vi "Zadanie 3.vi"() -> ()   [LabVIEW 2020]
doc: "Use this template to build a producer/consumer design pattern with events to produce queue items. Use this design pattern instead of the User Interface Event Handler pattern for user interfaces when you want to execute code asynchronously in response to an event without slowing the user interface responsiveness."
panel:
  out "Waveform Graph":dbl[](graph)
  in  "What to add?":dbl
  out "Busy":bool
  in  "?":bool
  out "Generated numbers":dbl[](array[numeric])
  in  "?":bool
  in  "REMOVE":bool
  in  "stop":bool
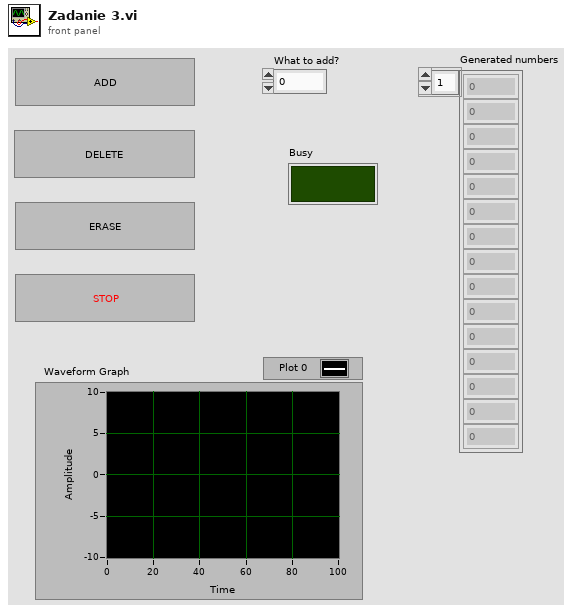
[diagram p1: front panel]
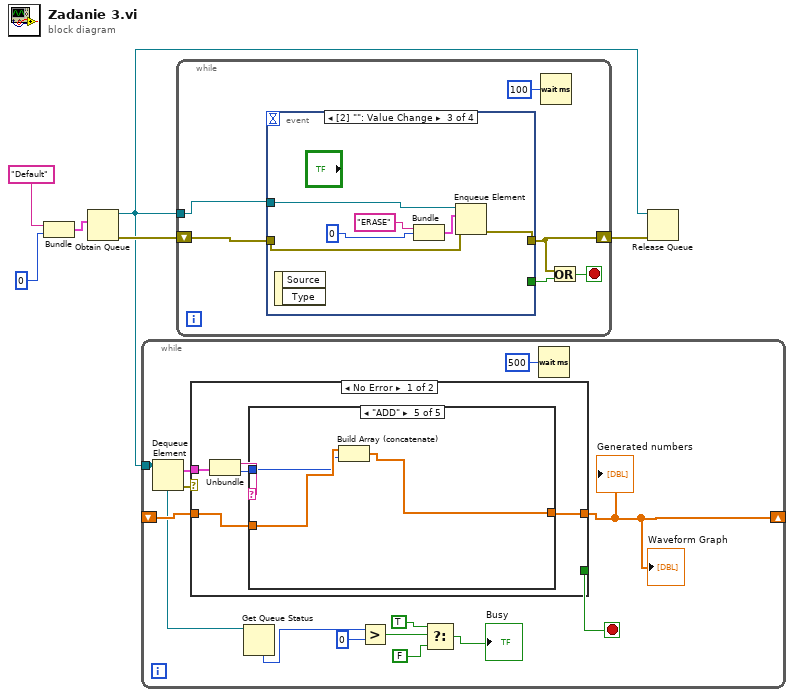
[diagram p0: block diagram]
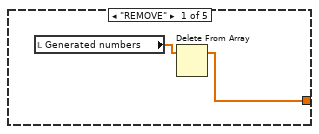
[diagram p2: hidden frame]
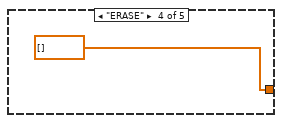
[diagram p5: hidden frame]
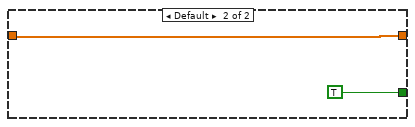
[diagram p6: hidden frame]
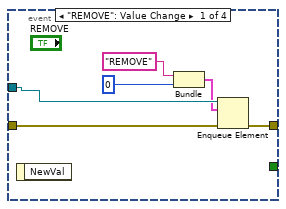
[diagram p7: hidden frame]
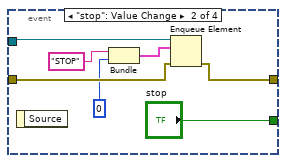
[diagram p8: hidden frame]
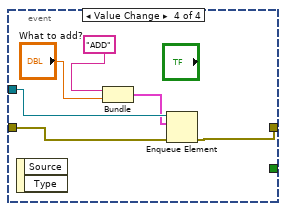
[diagram p9: hidden frame]
diagram:
  n1 = Bundle("Default", 0) -> (w2:cluster{string, i32})  [unwired: 1 in]
  n2 = Obtain Queue(element data type=w2) -> (queue out=w4:refnum<queue>, error out=w6:errorcluster)  [unwired: 4 in, 1 out]
  n3 = while {
    tunnel: w4 -> [w14]
    shift-right: [w7] -> _
    shift-left: _ -> [w15]
    stop <- w17 stop-if-true
    n4 = Dequeue Element(queue=w14) -> (element=w18:cluster{string, i32}, error out=w19:errorcluster)  [unwired: 2 in, 2 out]
    n5 = case shown="No Error" w19 {
      tunnel: w18 -> [w20 _]
      tunnel: [_ TRUE] -> w17
      tunnel: w15 -> [w24 w33]
      tunnel: [w23 w33] -> w7
      frame No Error {
        n6 = Unbundle(w20) -> (w22:string, w21:i32)
        n7 = case shown="\"ADD\"" w22 {
          tunnel: [w25 w27 w28 dbl[] [] w31] -> w23
          tunnel: w24 -> [_ w27 w28 _ w32]
          tunnel: w21 -> [_ _ _ _ w30]
          frame "REMOVE" {
            n8 = local read "Generated numbers"() -> (w26:dbl[])
            n9 = Delete From Array(array=w26) -> (array with subset deleted=w25:dbl[])  [unwired: 2 in, 1 out]
          }
          frame "STOP" {
          }
          frame Default {
          }
          frame "ERASE" {
          }
          frame "ADD" {
            n10 = Build Array (concatenate)(w32, w30) -> (w31:dbl[])
          }
        }
      }
      frame Default {
      }
    }
    "Generated numbers" <- w7
    "Waveform Graph" <- w7
    n11 = Get Queue Status(queue=w14) -> (# elements in queue=w13:i32)  [unwired: 2 in, 7 out]
    n12 = Greater?(x=w13, y=0) -> (0:w11:bool)
    n13 = Select(t=TRUE, s=w11, f=FALSE) -> (s? t:f=→"Busy":bool)
    n14 = Wait (ms)(milliseconds to wait=u32 500) -> ()  [unwired: 1 out]
  }
  n15 = while {
    shift-right: [w37] -> w5
    shift-left: w6 -> [w40]
    tunnel: w4 -> [w35]
    stop <- w38 stop-if-true
    n16 = event shown="[2] \"\": Value Change" {
      selector: _ -> [_ _ _ _]
      dyn-events: _ -> [_ _ _ _]
      timeout: _ -> [_ _ _ _]
      tunnel: w40 -> [w46 w52 w59 w65]
      tunnel: [w45 w51 w58 w64] -> w37
      tunnel: [_ "stop" _ _] -> w39
      tunnel: w35 -> [w44 w50 w57 w63]
      event "REMOVE": Value Change {
        n17 = event-data() -> ()  [unwired: 1 in, 1 out]
        n18 = Bundle("REMOVE", 0) -> (w41:cluster{string, i32})  [unwired: 1 in]
        n19 = Enqueue Element(queue=w44, element=w41, error in (no error)=w46) -> (error out=w45:errorcluster)  [unwired: 1 in, 2 out]
      }
      event "stop": Value Change {
        n20 = event-data() -> ()  [unwired: 1 in, 1 out]
        n21 = Bundle("element"="STOP", 0) -> (w48:cluster{"element":string, i32})  [unwired: 1 in]
        n22 = Enqueue Element(queue=w50, element=w48, error in (no error)=w52) -> (error out=w51:errorcluster)  [unwired: 1 in, 2 out]
      }
      event Value Change {
        n23 = event-data() -> ()  [unwired: 1 in, 2 out]
        n24 = Bundle("element"="ERASE", 0) -> (w55:cluster{"element":string, i32})  [unwired: 1 in]
        n25 = Enqueue Element(queue=w57, element=w55, error in (no error)=w59) -> (error out=w58:errorcluster)  [unwired: 1 in, 2 out]
      }
      event Value Change {
        n26 = event-data() -> ()  [unwired: 1 in, 2 out]
        n27 = Bundle("ADD", "What to add?"="What to add?") -> (w62:cluster{string, "What to add?":dbl})  [unwired: 1 in]
        n28 = Enqueue Element(queue=w63, element=w62, error in (no error)=w65) -> (error out=w64:errorcluster)  [unwired: 1 in, 2 out]
      }
    }
    n29 = Wait (ms)(milliseconds to wait=u32 100) -> ()  [unwired: 1 out]
    n30 = Or(x=w37, y=w39) -> (x .or. y?=w38:bool)
  }
  n31 = Release Queue(queue=w4, error in (no error)=w5) -> ()  [unwired: 1 in, 3 out]
